vi "HMI wrapper.vi"(6 "Process State":u16(ring)=1, 8 "Elapsed time in current state":dbl format="%.2f", 9 "Current Control settings":T1 {"fractional duty" format="%#_3g"}, 10 "smooth interval (s)":sgl format="%.3f", 11 "HMI panel":T2) -> (0 "error out":errorcluster)   [LabVIEW 2010]
uses:
  DAQ configuration/Sensor buffer command.ctl
  logic buffer cmd.ctl
  HMI VI type.ctl
  switch and fraction.ctl
panel:
  in  "Control names":string[](array[string])=["Current Control settings", "Sensor Data smoothed", "Set Points", "Elapsed time in current state", "Process State"]
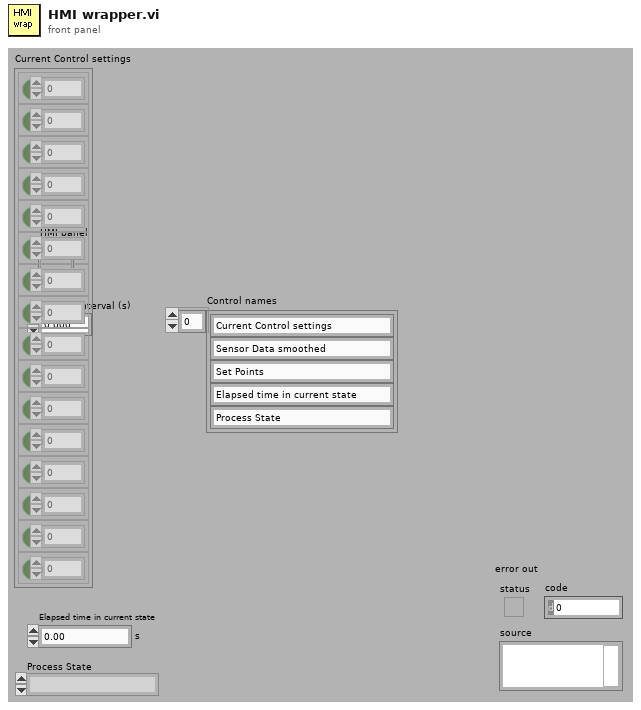
[diagram p1: front panel]
types:
  T1 = typedef "switch and fraction.ctl" = cluster{"switch":bool, "fractional duty":dbl}[]
  T2 = typedef "HMI VI type.ctl" = refnum<vi>
  T3 = typedef "logic buffer cmd.ctl" = enum16{"read", "write ouput settings", "write rules", "write setpoints", "write output descriptions", "write all", "calculate setpoints", "save", "open", "Load all setpoint code", "Load one setpoint code"}
  T4 = typedef "Sensor buffer command.ctl" = enum16{"read average", "read recent", "read all", "write", "configure", "clear"}
  T5 = typedef "rules.ctl" = T6[]
  T6 = typedef "State rules.ctl" = cluster{"state rules":T7[], "State name":string}
  T7 = typedef "rule.ctl" = cluster{"next state":u16, "conditions":T8[], "number of conditions":u8, "Rule name":string}
  T8 = typedef "condition.ctl" = cluster{"> or <":T9, "set point":i32, "sensor data":i32, "Data average interval":dbl}
  T9 = typedef "greater or less.ctl" = bool
  T10 = typedef "Set Points.ctl" = cluster{"name":string, "unit":string, "value":dbl}
  T11 = typedef "Sensor data.ctl" = cluster{" Sensor array":T12[], "Time":dbl}
  T12 = typedef "sensor cluster.ctl" = cluster{"voltage":sgl, "scaled":sgl, "units":string, "Out of Range":bool}
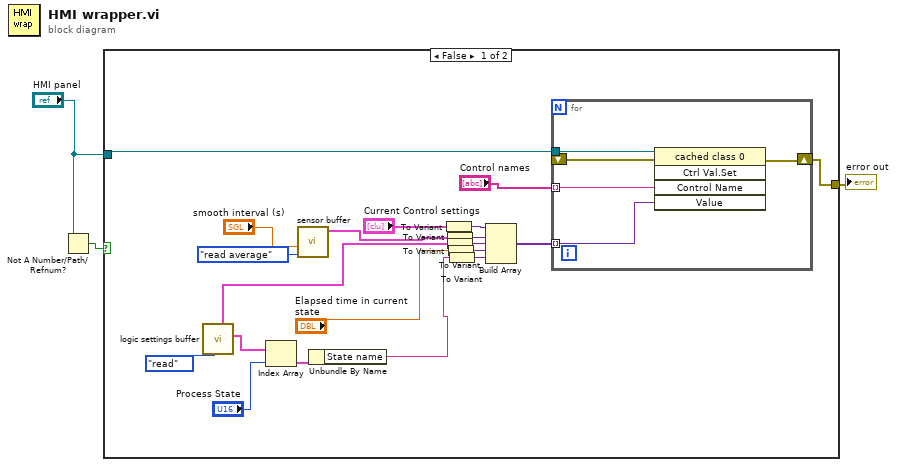
[diagram p0: block diagram]
diagram:
  n1 = Not A Number/Path/Refnum?(number/path/refnum="HMI panel") -> (NaN/Path/Refnum?=w1:bool)
  n2 = case shown="False" w1 {
    tunnel: "HMI panel" -> [w7 _]
    tunnel: [w4 _] -> w2
    frame False {
      n3 = call "logic settings buffer.vi"("command"=logic_buffer_cmd."read") -> ("Rules out"=w12:T5, "Set Points out"=w10:T10[])  [unwired: 6 in, 3 out]
      n4 = Index Array(array=w12, index="Process State") -> (element=w14:T6)
      n5 = call "sensor buffer.vi"("command"=Sensor_buffer_command."read average", "smooth interval (s)"="smooth interval (s)") -> ("Sensor Data smoothed"=w15:T11)  [unwired: 3 in, 2 out]
      n6 = Unbundle By Name(w14) -> ("State name"=w8:string)
      n7 = To Variant(anything="Current Control settings") -> (Variant=w23:variant)
      n8 = To Variant(anything=w15) -> (Variant=w21:variant)
      n9 = To Variant(anything=w10) -> (Variant=w20:variant)
      n10 = To Variant(anything="Elapsed time in current state") -> (Variant=w19:variant)
      n11 = To Variant(anything=w8) -> (Variant=w18:variant)
      n12 = Build Array(w23, w21, w20, w19, w18) -> (w5:variant[])
      n13 = for {
        tunnel: w7 -> [w28]
        tunnel: "Control names" -> [w27] mode=indexing
        tunnel: w5 -> [w26] mode=indexing
        shift-right: [w25] -> w4
        shift-left: _ -> [w24]
        n14 = invoke class="cached class 0" method="Ctrl Val.Set"(reference=w28, error in=w24, "Control Name"=w27, "Value"=w26) -> (error out=w25:errorcluster)  [unwired: 1 in, 4 out]
      }
    }
    frame True {
    }
  }
  "error out" <- w2
